vi "MFC.vi"(0 "MFC":string(combo)="42", 5 "Set Point\n(SCCM)":dbl(knob) min=0.0 max=500.0 step=1.0 scale=0.0..500.0) -> (4 "Flow\n(SCCM)":dbl(knob) scale=-25.0..665.0, 6 "Set Point 2\n(SCCM)":dbl(knob) scale=0.0..550.0)   [LabVIEW 2011]
panel:
  out "MFC/PC?":string="MFC"
  out "SCCM":dbl=500.0
  in  "stop":bool
  in  "Full Scale":dbl=24576.0
  out "Set Point\n(%)":dbl(slide) scale=0.0..110.0
  out "Flow\n(%)":dbl(slide) scale=0.0..140.0
  out "Actuator Drive Value":i16
  out "Actuator Override":i8
  out "Manufacturer Specific Warnings":bool caption="Boolean"
  out "Device Profice Specific Warnings":bool caption="Boolean"
  out "Common Warnings":bool caption="Boolean"
  out "0":bool caption="Boolean"
  out "Manufactuer Specific Alarms":bool caption="Boolean"
  out "1 (Extended Reporting Enabled)":bool caption="Boolean"
  out "Device Profile Specific Alarms":bool caption="Boolean"
  out "Common Alarms":bool caption="Boolean"
  # "0    -  24576\n   0% to  100%\n\n\n 24577  - 27033\n100+% to 110%\n\n\n 27034  -  32767\n110+% to 133%"
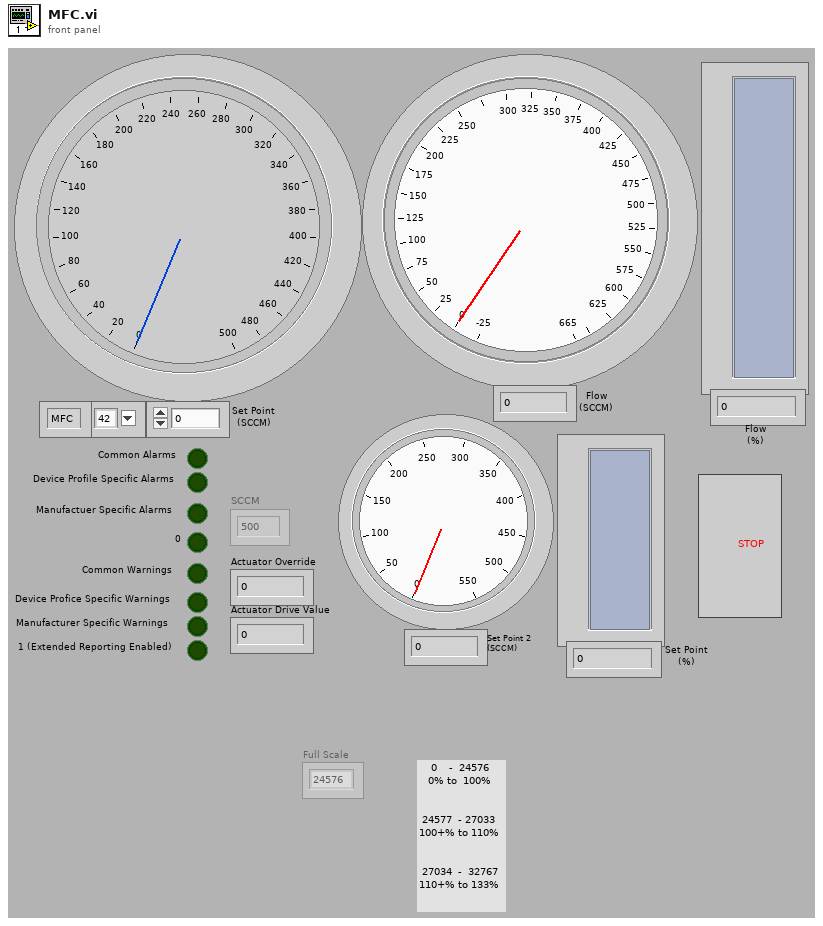
[diagram p1: front panel]
types:
  T1 = enum16{"No dialog", "OK message", "Continue or stop message", "OK message with warnings", "Continue or stop message with warnings"}
  T2 = enum16{"Read", "Write", "ReadWrite", "BufferedRead", "BufferedReadWrite"}
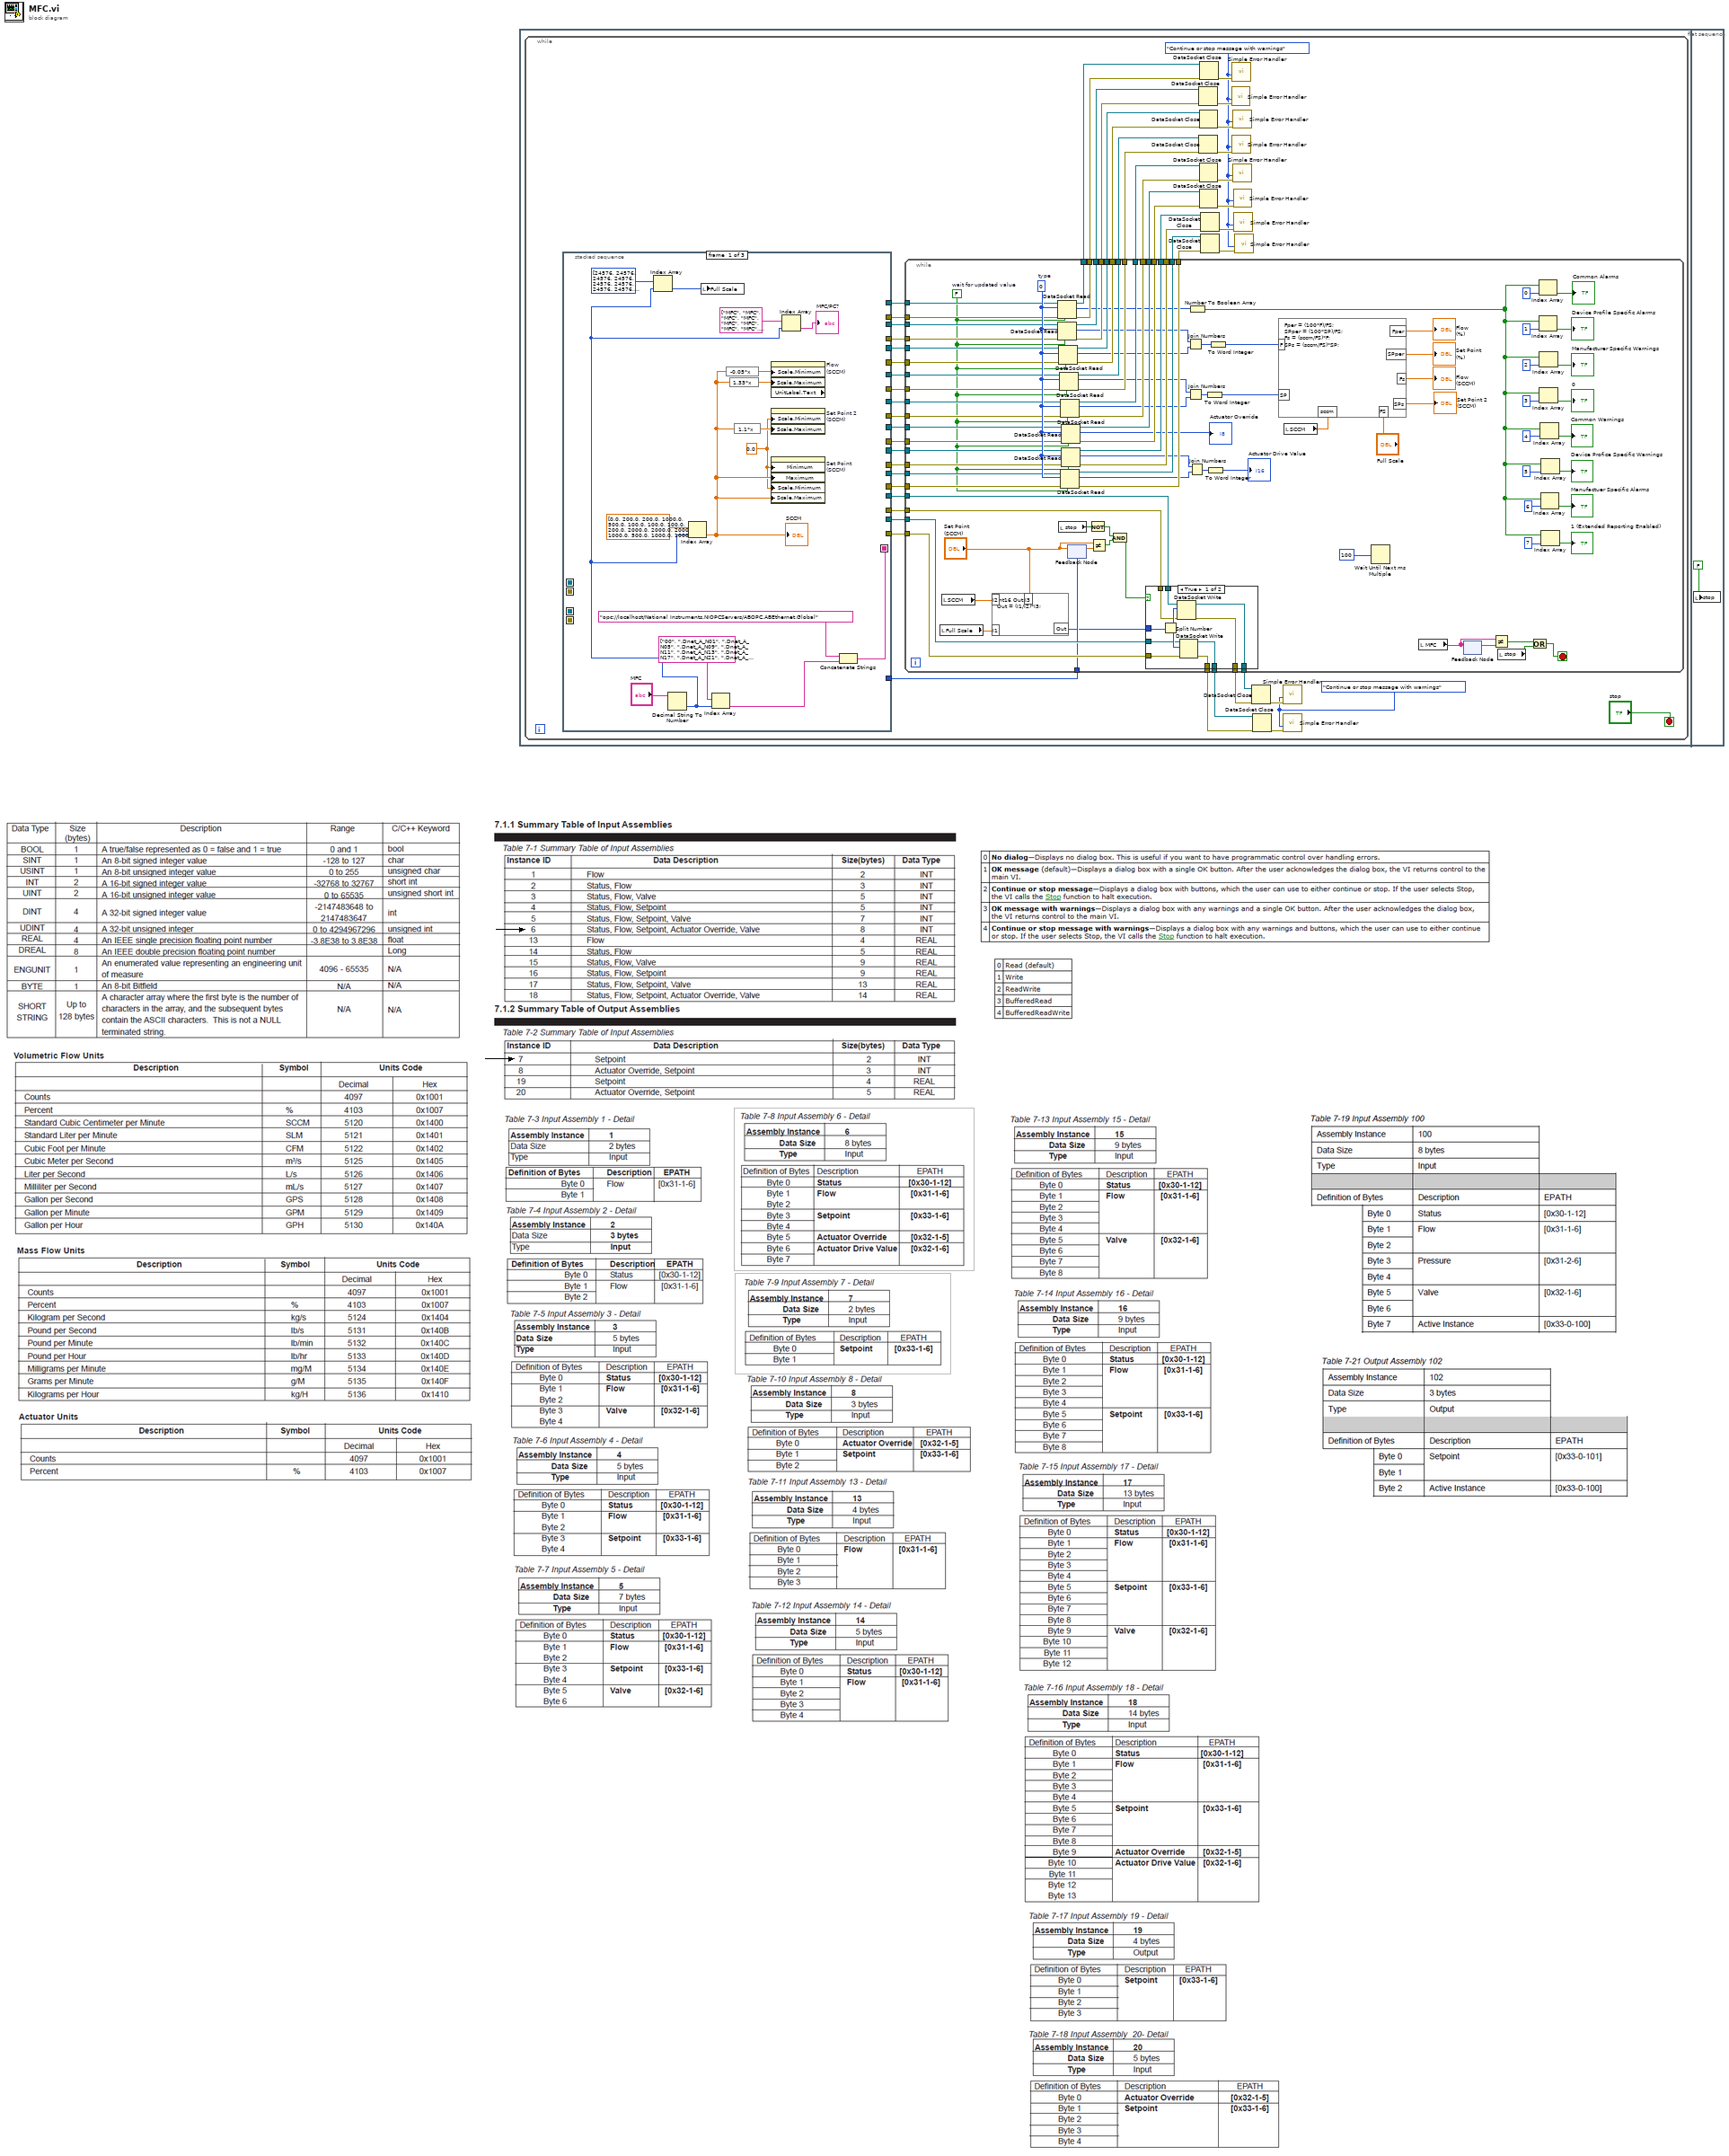
[diagram p0: block diagram]
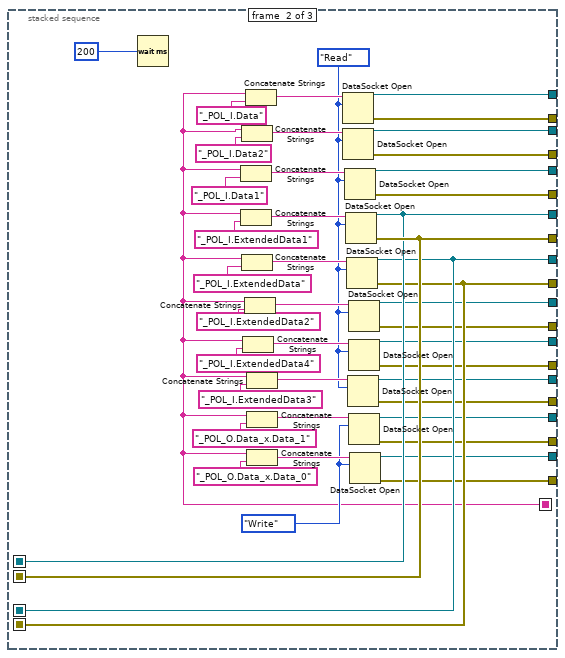
[diagram p2: hidden frame]
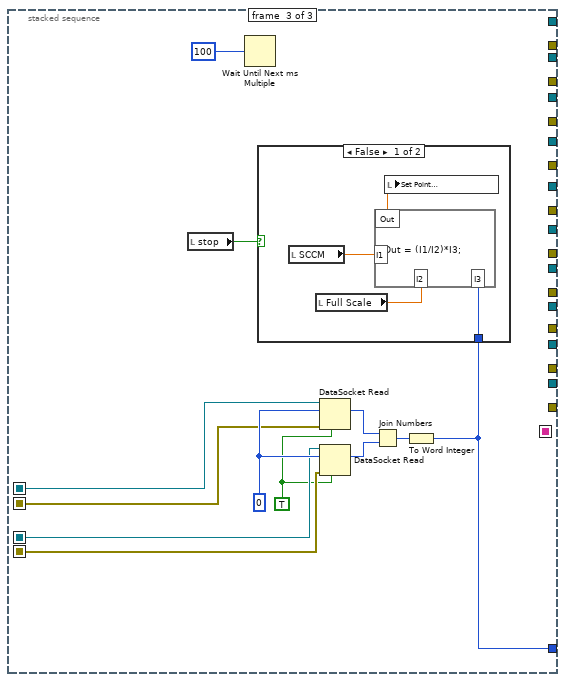
[diagram p3: hidden frame]
diagram:
  n1 = flat-sequence {
    frame #0 {
      n2 = while {
        stop <- "stop" stop-if-true
        w6 = T1."Continue or stop message with warnings"
        w29 = T1."Continue or stop message with warnings"
        n3 = stacked-sequence {
          seq-local: [_ w114 _] -> [_ _ w122]
          seq-local: [_ w113 _] -> [_ _ w119]
          seq-local: [_ w111 _] -> [_ _ w121]
          seq-local: [_ w112 _] -> [_ _ w120]
          seq-local: [w67 _ _] -> [_ w71 _]
          tunnel: [_ w113 _] -> w54
          tunnel: [_ w114 _] -> w53
          tunnel: [_ w112 _] -> w52
          tunnel: [_ w111 _] -> w51
          tunnel: [_ w81 _] -> w49
          tunnel: [_ w80 _] -> w48
          tunnel: [_ w79 _] -> w47
          tunnel: [_ w78 _] -> w46
          tunnel: [_ w77 _] -> w45
          tunnel: [_ w76 _] -> w44
          tunnel: [_ w92 _] -> w43
          tunnel: [_ w91 _] -> w42
          tunnel: [_ w90 _] -> w41
          tunnel: [_ w89 _] -> w40
          tunnel: [_ w88 _] -> w39
          tunnel: [_ w87 _] -> w38
          tunnel: [_ w75 _] -> w5
          tunnel: [_ w72 _] -> w4
          tunnel: [_ w74 _] -> w3
          tunnel: [_ w73 _] -> w2
          tunnel: [_ _ w117] -> w1
          frame #0 {
            w60 = 0.0
            n4 = Decimal String To Number(string="MFC") -> (number=w56:i32)  [unwired: 2 in, 1 out]
            n5 = Index Array(array=i16[] [24576, 24576, 24576, 24576, 24576, 24576, 24576, 24576, 24576, 24576, 24576, 24576, 24576, 24576, 24576, 24576, 24576, 24576, 24576, 24576, 24576, 24576, 24576, 24576, 24576, 24576, 24576, 24576, 24576, 24576, 24576, 24576, 24576, 24576, 24576, 24576, 24576, 24576, 24576, 24576, 24576, 24576, 24576, 24576, 24576, 24576, 24576, 24576, 24576, 24576, 24576, 24576, 24576, 24576, 24576, 24576, 24576, 24576, 24576, 24576, 24576, 24576, 24576, 24576, 24576, 24576, 24576, 24576, 24576, 24576, 24576, 24576, 24576, 24576, 24576, 24576, 24576, 24576, 24576, 24576, 24576, 24576, 24576, 24576, 24576, 24576, 24576], index=w56) -> (element=w55:i16)
            n6 = Index Array(array=dbl[] [0.0, 200.0, 200.0, 1000.0, 500.0, 100.0, 100.0, 100.0, 200.0, 2000.0, 2000.0, 2000.0, 1000.0, 500.0, 1000.0, 1000.0, 1000.0, 1000.0, 0.0, 1000.0, 100.0, 1000.0, 2000.0, 1000.0, 2000.0, 0.0, 0.0, 5000.0, 5000.0, 5000.0, 5000.0, 0.0, 100.0, 1000.0, 2000.0, 2000.0, 100.0, 100.0, 2000.0, 100.0, 0.0, 10.0, 500.0, 500.0, 2000.0, 200.0, 2000.0, 200.0, 1000.0, 100.0, 1000.0, 100.0, 1000.0, 100.0, 2000.0, 200.0, 500.0, 1000.0, 0.0, 0.0, 0.0, 0.0, 0.0, 0.0, 0.0, 0.0, 0.0, 0.0, 2000.0, 2000.0, 500.0, 0.0, 0.0, 1000.0, 1000.0, 5000.0, 0.0, 0.0, 2000.0, 2000.0, 2000.0, 20000.0, 20000.0, 20000.0, 1000.0, 1000.0, 2000.0], index=w56) -> (element=w62:dbl)
            "SCCM" <- w62
            n7 = local write "Full Scale"(w55) -> ()
            n8 = Index Array(array=string[] ["00", ".Dnet_A_N01", ".Dnet_A_N05", ".Dnet_A_N09", ".Dnet_A_N11", ".Dnet_A_N13", ".Dnet_A_N17", ".Dnet_A_N21", ".Dnet_A_N25", "00", ".Dnet_A_N04", ".Dnet_A_N08", ".Dnet_A_N10", ".Dnet_A_N12", ".Dnet_A_N14", ".Dnet_A_N20", ".Dnet_A_N24", ".Dnet_A_N28", "00", "00", "00", "00", "00", "00", "00", "00", "00", "00", "00", "00", "00", "00", "00", "00", "00", "00", "00", ".Dnet_A_N31", "00", "00", "00", ".Dnet_A_N56", ".Dnet_A_N42", "00", ".Dnet_A_N02", ".Dnet_A_N03", ".Dnet_A_N06", ".Dnet_A_N07", ".Dnet_A_N14", ".Dnet_A_N15", ".Dnet_A_N50", ".Dnet_A_N19", ".Dnet_A_N37", ".Dnet_A_N23", ".Dnet_A_N51", ".Dnet_A_N27", ".Dnet_A_N32", ".Dnet_A_N55", "00", "00", "00", "00", "00", "00", "00", "00", "00", "00", ".Dnet_B_N08", ".Dnet_B_N10", ".Dnet_B_N12", "00", "00", ".Dnet_B_N13", ".Dnet_B_N14", ".Dnet_B_N15", "00", "00", ".Dnet_B_N01", ".Dnet_B_N02", ".Dnet_B_N03", ".Dnet_B_N05", ".Dnet_B_N06", ".Dnet_B_N04", "00", ".Dnet_B_N09", ".Dnet_B_N11"], index=w56) -> (element=w68:string)
            n9 = expression code="-0.05*x"(w62) -> (w63:dbl)
            n10 = expression code="1.33*x"(w62) -> (w64:dbl)
            n11 = expression code="1.1*x"(w62) -> (w61:dbl)
            n12 = property on="Flow\n(SCCM)" class="Knob (strict)" props=["Scale", "Minimum", "Scale", "Maximum", "UnitLabel", "Text"]("Scale.Minimum"=w63, "Scale.Maximum"=w64) -> ()  [unwired: 2 in, 3 out]
            n13 = property on="Set Point 2\n(SCCM)" class="Knob (strict)"("Scale.Minimum"=w60, "Scale.Maximum"=w61) -> ()  [unwired: 2 in, 2 out]
            n14 = property on="Set Point\n(SCCM)" class="Knob (strict)"("Minimum"=w60, "Maximum"=w62, "Scale.Minimum"=w60, "Scale.Maximum"=w62) -> ()  [unwired: 2 in, 2 out]
            n15 = Index Array(array=string[] ["MFC", "MFC", "MFC", "MFC", "MFC", "MFC", "MFC", "MFC", "MFC", "MFC", "PC", "PC", "PC", "PC", "PC", "PC", "PC", "PC", "MFC", "MFC", "MFC", "MFC", "MFC", "MFC", "MFC", "MFC", "MFC", "MFC", "MFC", "MFC", "MFC", "MFC", "MFC", "MFC", "MFC", "MFC", "MFC", "MFC", "MFC", "MFC", "MFC", "MFC", "MFC", "MFC", "MFC", "MFC", "MFC", "MFC", "MFC", "MFC", "MFC", "MFC", "MFC", "MFC", "MFC", "MFC", "MFC", "MFC", "MFC", "MFC", "MFC", "MFC", "MFC", "MFC", "MFC", "MFC", "MFC", "MFC", "MFC", "MFC", "MFC", "MFC", "MFC", "MFC", "MFC", "MFC", "MFC", "MFC", "MFC", "MFC", "MFC", "MFC", "MFC", "MFC", "MFC", "MFC", "MFC"], index=w56) -> (element=→"MFC/PC?":string)
            n16 = Concatenate Strings("opc://localhost/National Instruments.NIOPCServers/ABOPC.ABEthernet.Global", w68) -> (w67:string)
          }
          frame #1 {
            w83 = T2."Write" ("mode")
            w86 = T2."Read" ("mode")
            n17 = Wait (ms)(milliseconds to wait=u32 200) -> ()  [unwired: 1 out]
            n18 = Concatenate Strings(w71, "_POL_I.Data1") -> (w98:string)
            n19 = Concatenate Strings(w71, "_POL_I.ExtendedData1") -> (w97:string)
            n20 = Concatenate Strings(w71, "_POL_I.Data2") -> (w99:string)
            n21 = Concatenate Strings(w71, "_POL_I.ExtendedData") -> (w96:string)
            n22 = Concatenate Strings(w71, "_POL_I.ExtendedData4") -> (w94:string)
            n23 = Concatenate Strings(w71, "_POL_I.ExtendedData2") -> (w95:string)
            n24 = Concatenate Strings(w71, "_POL_I.Data") -> (w100:string)
            n25 = Concatenate Strings(w71, "_POL_I.ExtendedData3") -> (w93:string)
            n26 = Concatenate Strings(w71, "_POL_O.Data_x.Data_1") -> (w84:string)
            n27 = Concatenate Strings(w71, "_POL_O.Data_x.Data_0") -> (w85:string)
            n28 = DataSocket Open(10:w86, 11:w100) -> (0:w88:errorcluster, 3:w87:refnum<k13>)  [unwired: 2 in]
            n29 = DataSocket Open(10:w86, 11:w99) -> (0:w90:errorcluster, 3:w89:refnum<k13>)  [unwired: 2 in]
            n30 = DataSocket Open(10:w86, 11:w98) -> (0:w92:errorcluster, 3:w91:refnum<k13>)  [unwired: 2 in]
            n31 = DataSocket Open(10:w86, 11:w97) -> (0:w114:errorcluster, 3:w113:refnum<k13>)  [unwired: 2 in]
            n32 = DataSocket Open(10:w86, 11:w96) -> (0:w111:errorcluster, 3:w112:refnum<k13>)  [unwired: 2 in]
            n33 = DataSocket Open(10:w86, 11:w93) -> (0:w80:errorcluster, 3:w81:refnum<k13>)  [unwired: 2 in]
            n34 = DataSocket Open(10:w86, 11:w95) -> (0:w77:errorcluster, 3:w76:refnum<k13>)  [unwired: 2 in]
            n35 = DataSocket Open(10:w86, 11:w94) -> (0:w79:errorcluster, 3:w78:refnum<k13>)  [unwired: 2 in]
            n36 = DataSocket Open(10:w83, 11:w84) -> (0:w72:errorcluster, 3:w75:refnum<k13>)  [unwired: 2 in]
            n37 = DataSocket Open(10:w83, 11:w85) -> (0:w73:errorcluster, 3:w74:refnum<k13>)  [unwired: 2 in]
          }
          frame #2 {
            w118 = TRUE
            w123 = i8 0
            n38 = local read "stop"() -> (w116:bool)
            n39 = Wait Until Next ms Multiple(millisecond multiple=u32 100) -> ()  [unwired: 1 out]
            n40 = DataSocket Read(6:w118, 8:w122, 10:w123, 11:w119) -> (2:w125:i8)  [unwired: 1 in, 6 out]
            n41 = DataSocket Read(6:w118, 8:w121, 10:w123, 11:w120) -> (2:w126:i8)  [unwired: 1 in, 6 out]
            n42 = Join Numbers(hi=w125, lo=w126) -> ((hi.lo)=w124:u16)
            n43 = To Word Integer(number=w124) -> (16bit integer=w117:i16)
            n44 = case shown="False" w116 {
              tunnel: w117 -> [w127 _]
              frame False {
                n45 = local read "SCCM"() -> (w128:dbl)
                n46 = local read "Full Scale"() -> (w130:dbl)
                n47 = formula code="Out = (I1/I2)*I3;"("I1"=w128, "I2"=w130, "I3"=w127) -> ("Out"=w129:dbl)
                n48 = local write "Set Point\n(SCCM)"(w129) -> ()
              }
              frame True {
              }
            }
          }
        }
        n49 = while {
          tunnel: w49 -> [w200]
          tunnel: w48 -> [w199]
          tunnel: w47 -> [w198]
          tunnel: w46 -> [w197]
          tunnel: w45 -> [w196]
          tunnel: w44 -> [w195]
          tunnel: w51 -> [w194]
          tunnel: w52 -> [w193]
          tunnel: w53 -> [w192]
          tunnel: w54 -> [w191]
          tunnel: w43 -> [w190]
          tunnel: w42 -> [w189]
          tunnel: w41 -> [w188]
          tunnel: w40 -> [w187]
          tunnel: w39 -> [w186]
          tunnel: w38 -> [w185]
          tunnel: [w184] -> w28
          tunnel: [w183] -> w27
          tunnel: [w182] -> w26
          tunnel: [w181] -> w25
          tunnel: [w180] -> w24
          tunnel: [w179] -> w23
          tunnel: [w178] -> w22
          tunnel: [w177] -> w21
          tunnel: [w176] -> w20
          tunnel: [w175] -> w19
          tunnel: [w174] -> w18
          tunnel: [w173] -> w17
          tunnel: [w172] -> w16
          tunnel: [w171] -> w15
          tunnel: [w170] -> w14
          tunnel: [w169] -> w13
          tunnel: [w166] -> w10
          tunnel: [w165] -> w9
          tunnel: [w164] -> w8
          tunnel: [w163] -> w7
          tunnel: w5 -> [w162]
          tunnel: w4 -> [w161]
          tunnel: w3 -> [w160]
          tunnel: w2 -> [w159]
          tunnel: w1 -> [w158]
          stop <- w203 stop-if-true
          w167 = FALSE  # wait for updated value
          w225 = i8 0  # type
          n50 = local read "Full Scale"() -> (w143:dbl)
          n51 = local read "SCCM"() -> (w139:dbl)
          n52 = formula code="int16 Out;\nOut = (I1/I2)*I3;"("I3"="Set Point\n(SCCM)", "I1"=w143, "I2"=w139) -> ("Out"=w142:i16)
          n53 = DataSocket Read(6:w167, 8:w186, 10:w225, 11:w185) -> (0:w180:errorcluster, 2:w145:i8, 3:w181:refnum<k13>)  [unwired: 1 in, 4 out]
          n54 = DataSocket Read(6:w167, 8:w188, 10:w225, 11:w187) -> (0:w178:errorcluster, 2:w146:i8, 3:w179:refnum<k13>)  [unwired: 1 in, 4 out]
          n55 = DataSocket Read(6:w167, 8:w190, 10:w225, 11:w189) -> (0:w176:errorcluster, 2:w147:i8, 3:w177:refnum<k13>)  [unwired: 1 in, 4 out]
          n56 = local read "stop"() -> (w156:bool)
          n57 = DataSocket Read(6:w167, 8:w192, 10:w225, 11:w191) -> (0:w174:errorcluster, 2:w148:i8, 3:w175:refnum<k13>)  [unwired: 1 in, 4 out]
          n58 = DataSocket Read(6:w167, 8:w194, 10:w225, 11:w193) -> (0:w171:errorcluster, 2:w149:i8, 3:w169:refnum<k13>)  [unwired: 1 in, 4 out]
          n59 = DataSocket Read(6:w167, 8:w199, 10:w225, 11:w200) -> (0:w184:errorcluster, 2:w152:i8, 3:w183:refnum<k13>)  [unwired: 1 in, 4 out]
          n60 = DataSocket Read(6:w167, 8:w196, 10:w225, 11:w195) -> (0:w173:errorcluster, 2:→"Actuator Override":i8, 3:w170:refnum<k13>)  [unwired: 1 in, 4 out]
          n61 = DataSocket Read(6:w167, 8:w198, 10:w225, 11:w197) -> (0:w182:errorcluster, 2:w151:i8, 3:w172:refnum<k13>)  [unwired: 1 in, 4 out]
          n62 = feedback #1(w158) -> (w157:dbl)
          n63 = feedback-in #1("Set Point\n(SCCM)") -> ()
          n64 = Not(x=w156) -> (.not. x?=w153:bool)
          n65 = Not Equal?(x="Set Point\n(SCCM)", y=w157) -> (x != y?=w154:bool)
          n66 = And(x=w153, y=w154) -> (x .and. y?=w155:bool)
          n67 = case shown="True" w155 {
            tunnel: w142 -> [w234 _]
            tunnel: [w233 w237] -> w166
            tunnel: [w232 w238] -> w165
            tunnel: [w231 w239] -> w164
            tunnel: [w230 w240] -> w163
            tunnel: w162 -> [w229 w240]
            tunnel: w161 -> [w228 w239]
            tunnel: w160 -> [w227 w238]
            tunnel: w159 -> [w226 w237]
            frame True {
              n68 = Split Number(x=w234) -> (hi(x)=w236:u8, lo(x)=w235:u8)
              n69 = DataSocket Write(8:w228, 10:w236, 11:w229) -> (0:w231:errorcluster, 3:w230:refnum<k13>)  [unwired: 1 in, 1 out]
              n70 = DataSocket Write(8:w226, 10:w235, 11:w227) -> (0:w233:errorcluster, 3:w232:refnum<k13>)  [unwired: 1 in, 1 out]
            }
            frame False {
            }
          }
          n71 = Join Numbers(hi=w146, lo=w147) -> ((hi.lo)=w207:u16)
          n72 = Join Numbers(hi=w148, lo=w149) -> ((hi.lo)=w208:u16)
          n73 = Join Numbers(hi=w151, lo=w152) -> ((hi.lo)=w141:u16)
          n74 = Number To Boolean Array(number=w145) -> (Boolean array=w206:bool[])
          n75 = To Word Integer(number=w208) -> (16bit integer=w137:i16)
          n76 = To Word Integer(number=w141) -> (16bit integer=→"Actuator Drive Value":i16)
          n77 = To Word Integer(number=w207) -> (16bit integer=w138:i16)
          n78 = local read "SCCM"() -> (w136:dbl)
          n79 = formula code="Fper = (100*F)/FS;\nSPper = (100*SP)/FS;\nFs = (sccm/FS)*F;\nSPs = (sccm/FS)*SP;"("FS"="Full Scale", "F"=w138, "SP"=w137, "sccm"=w136) -> ("Fper"=→"Flow\n(%)":dbl, "SPper"=→"Set Point\n(%)":dbl, "Fs"=→"Flow\n(SCCM)":dbl, "SPs"=→"Set Point 2\n(SCCM)":dbl)
          n80 = Wait Until Next ms Multiple(millisecond multiple=u32 100) -> ()  [unwired: 1 out]
          n81 = local read "MFC"() -> (w201:string)
          n82 = feedback #2() -> (w205:string)  [unwired: 1 in]
          n83 = feedback-in #2(w201) -> ()
          n84 = Not Equal?(x=w201, y=w205) -> (x != y?=w204:bool)
          n85 = local read "stop"() -> (w202:bool)
          n86 = Or(x=w204, y=w202) -> (x .or. y?=w203:bool)
          n87 = Index Array(array=w206, index=0) -> (element=→"Common Alarms":bool)
          n88 = Index Array(array=w206, index=1) -> (element=→"Device Profile Specific Alarms":bool)
          n89 = Index Array(array=w206, index=2) -> (element=→"Manufacturer Specific Warnings":bool)
          n90 = Index Array(array=w206, index=3) -> (element=→"0":bool)
          n91 = Index Array(array=w206, index=4) -> (element=→"Common Warnings":bool)
          n92 = Index Array(array=w206, index=6) -> (element=→"Manufactuer Specific Alarms":bool)
          n93 = Index Array(array=w206, index=5) -> (element=→"Device Profice Specific Warnings":bool)
          n94 = Index Array(array=w206, index=7) -> (element=→"1 (Extended Reporting Enabled)":bool)
        }
        n95 = DataSocket Close(8:w22, 11:w23) -> (0:w31:errorcluster)  [unwired: 1 in, 1 out]
        n96 = DataSocket Close(8:w18, 11:w19) -> (0:w33:errorcluster)  [unwired: 1 in, 1 out]
        n97 = DataSocket Close(8:w20, 11:w21) -> (0:w32:errorcluster)  [unwired: 1 in, 1 out]
        n98 = DataSocket Close(8:w15, 11:w13) -> (0:w34:errorcluster)  [unwired: 1 in, 1 out]
        n99 = DataSocket Close(8:w17, 11:w14) -> (0:w35:errorcluster)  [unwired: 1 in, 1 out]
        n100 = DataSocket Close(8:w24, 11:w25) -> (0:w30:errorcluster)  [unwired: 1 in, 1 out]
        n101 = DataSocket Close(8:w26, 11:w16) -> (0:w36:errorcluster)  [unwired: 1 in, 1 out]
        n102 = DataSocket Close(8:w28, 11:w27) -> (0:w37:errorcluster)  [unwired: 1 in, 1 out]
        n103 = call <vilib>:"Simple Error Handler.vi"("type of dialog (OK msg:1)"=w29, "error in (no error)"=w31) -> ()  [unwired: 3 in, 5 out]
        n104 = call <vilib>:"Simple Error Handler.vi"("type of dialog (OK msg:1)"=w29, "error in (no error)"=w30) -> ()  [unwired: 3 in, 5 out]
        n105 = call <vilib>:"Simple Error Handler.vi"("type of dialog (OK msg:1)"=w29, "error in (no error)"=w33) -> ()  [unwired: 3 in, 5 out]
        n106 = call <vilib>:"Simple Error Handler.vi"("type of dialog (OK msg:1)"=w29, "error in (no error)"=w32) -> ()  [unwired: 3 in, 5 out]
        n107 = call <vilib>:"Simple Error Handler.vi"("type of dialog (OK msg:1)"=w29, "error in (no error)"=w34) -> ()  [unwired: 3 in, 5 out]
        n108 = call <vilib>:"Simple Error Handler.vi"("type of dialog (OK msg:1)"=w29, "error in (no error)"=w35) -> ()  [unwired: 3 in, 5 out]
        n109 = call <vilib>:"Simple Error Handler.vi"("type of dialog (OK msg:1)"=w29, "error in (no error)"=w36) -> ()  [unwired: 3 in, 5 out]
        n110 = call <vilib>:"Simple Error Handler.vi"("type of dialog (OK msg:1)"=w29, "error in (no error)"=w37) -> ()  [unwired: 3 in, 5 out]
        n111 = DataSocket Close(8:w8, 11:w7) -> (0:w11:errorcluster)  [unwired: 1 in, 1 out]
        n112 = DataSocket Close(8:w10, 11:w9) -> (0:w12:errorcluster)  [unwired: 1 in, 1 out]
        n113 = call <vilib>:"Simple Error Handler.vi"("type of dialog (OK msg:1)"=w6, "error in (no error)"=w11) -> ()  [unwired: 3 in, 5 out]
        n114 = call <vilib>:"Simple Error Handler.vi"("type of dialog (OK msg:1)"=w6, "error in (no error)"=w12) -> ()  [unwired: 3 in, 5 out]
      }
    }
    frame #1 {
      n115 = local write "stop"(FALSE) -> ()
    }
  }
